vi "SVT Crest Factor (1 Ch).vi"(6 "restart averaging (F)":bool, 8 "error in (no error)":errorcluster, 11 "scaled signal [EU]":waveform(dbl)) -> (0 "error out":errorcluster, 1 "RMS level [EU rms]":dbl=nan format="%.2f", 2 "peak level [EU]":dbl=nan format="%.2f", 3 "crest factor":dbl=nan format="%.2f")   [LabVIEW 2017]
doc: "Computes the crest factor, peak level, and RMS level of <B>scaled signal [EU]</B> or <B>even angle signal [EU]</B>. You can use this polymorphic VI to compute the crest factor for a single channel or for N channels, or for a single channel or N channels of resampled data. The data type you wire to the <B>scaled signal [EU]</B> or <B>even angle signal [EU]</B> input determines the polymorphic instance to use."
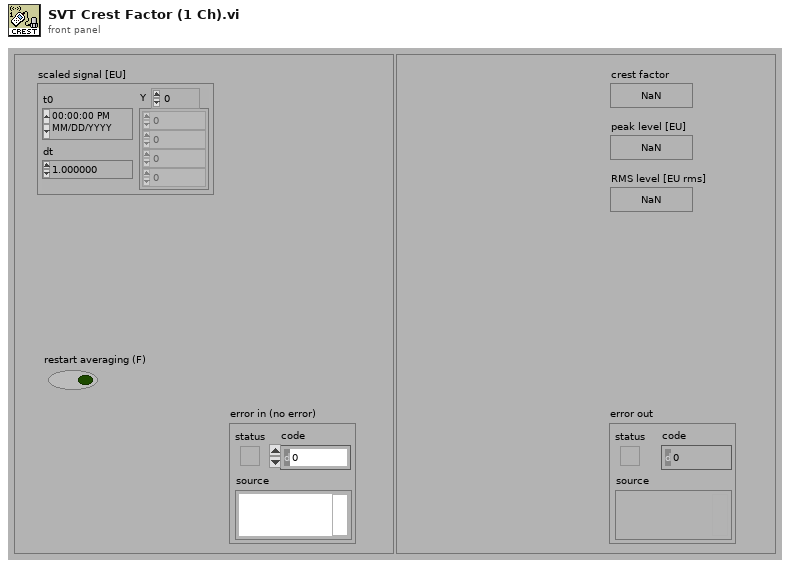
[diagram p1: front panel]
types:
  T1 = enum16{"RMS", "Running RMS", "Exp avg  ", "Dec exp avg ", "Peak", "Crest"}
  T2 = enum16{"Reset filter", "Restart averaging", "Continue processing"}
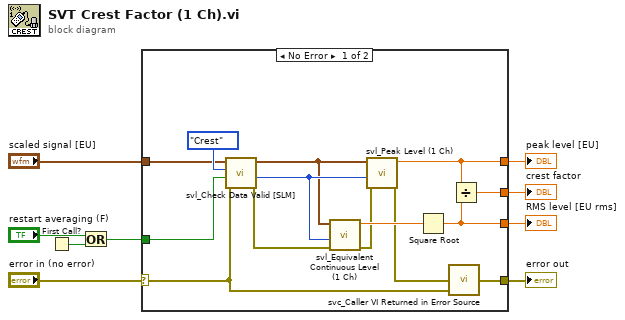
[diagram p0: block diagram]
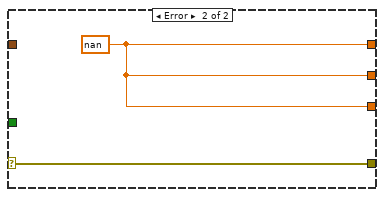
[diagram p2: hidden frame]
diagram:
  n1 = First Call?() -> (First Call?: T/F=w7:bool)
  n2 = Or(x="restart averaging (F)", y=w7) -> (x .or. y?=w6:bool)
  n3 = case shown="No Error" "error in (no error)" {
    tunnel: "scaled signal [EU]" -> [w13 _]
    tunnel: [w16 w24] -> w4
    tunnel: [w22 w24] -> w3
    tunnel: [w21 w24] -> w2
    tunnel: [w20 w25] -> w1
    tunnel: w6 -> [w19 _]
    selector: "error in (no error)" -> [w10 w25]
    frame No Error {
      n4 = call <vilib>:"svl_Check Data Valid [SLM].vi"("error in (no error)"=w10, "restart averaging (F)"=w19, "Level Analysis"=T1."Crest", "scaled signal [EU]"=w13) -> ("error out"=w12:errorcluster, "processing state"=w18:T2, "dup scaled signal [EU]"=w11:waveform(dbl))  [unwired: 4 in, 1 out]
      n5 = call <vilib>:"svl_Equivalent Continuous Level (1 Ch).vi"("error in (no error)"=w12, "processing state"=w18, "scaledSignal"=w11) -> ("error out"=w15:errorcluster, "equivalent continuous level [EU^2 rms]"=w23:dbl)  [unwired: 7 in]
      n6 = call <vilib>:"svl_Peak Level (1 Ch).vi"("error in (no error)"=w15, "processing state"=w18, "scaled signal"=w11) -> ("error out"=w14:errorcluster, "peak level"=w16:dbl)  [unwired: 7 in]
      n7 = Square Root(x=w23) -> (sqrt(x)=w21:dbl)
      n8 = call <vilib>:"svc_Caller VI Returned in Error Source.vi"("warning input to caller"=w10, "error in (no error)"=w14) -> ("error out"=w20:errorcluster)  [unwired: 3 in]
      n9 = Divide(x=w16, y=w21) -> (x/y=w22:dbl)
    }
    frame Error {
      w24 = nan
    }
  }
  "RMS level [EU rms]" <- w2
  "error out" <- w1
  "peak level [EU]" <- w4
  "crest factor" <- w3
